vi "String content_Str.vi"(4 "인덱스":i32, 6 "문자 배열":string[](array[string]), 7 "참조 배열":refnum<vi>[](array[refnum]), 8 "에러 입력":errorcluster caption="에러 입력(에러 없음)") -> (0 "에러 출력":errorcluster, 3 "참조":refnum<vi>)   [LabVIEW 2020]
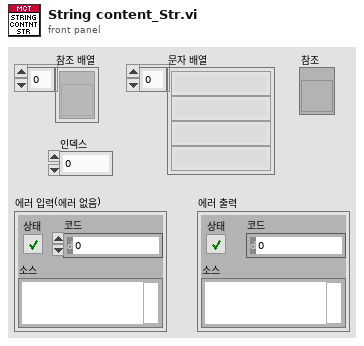
[diagram p1: front panel]
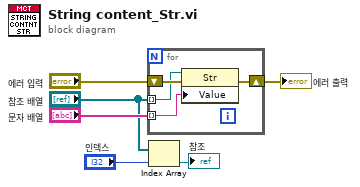
[diagram p0: block diagram]
diagram:
  n1 = for {
    shift-right: [w9] -> w5
    shift-left: "에러 입력" -> [w10]
    tunnel: "참조 배열" -> [w8] mode=indexing
    tunnel: "문자 배열" -> [w7] mode=indexing
    n2 = property class="Str"(reference=w8, error in=w10, "Value"=w7) -> (error out=w9:errorcluster)  [unwired: 1 out]
  }
  "에러 출력" <- w5
  n3 = Index Array(array="참조 배열", index="인덱스") -> (element=→"참조":refnum<vi>)
